vi "Insert Conditional.vi"(8 "error in (no error)":errorcluster, 10 "Insert Conditional":T1, 11 "Test Executive Builder Model in":refnum<class "Test Executive Builder Model.lvclass">) -> (0 "error out":errorcluster, 3 "Test Executive Builder Model out":refnum<class "Test Executive Builder Model.lvclass">, 5 "Unique ID out":string)   [LabVIEW 2017, in "Test Executive Builder Model.lvclass"]
uses:
  Test Executive Builder Model.lvclass
  <vilib>/gpm_packages/@cs/test-executive/Source/Test Executive/TestExecutive Ref/TestExecutive Ref.lvclass
  Test Executive Builder Model Messages/Redraw Tree Msg/Redraw Tree Msg.lvclass
  <vilib>/ActorFramework/Actor/Actor.lvclass
  <vilib>/gpm_packages/@cs/run-time-assertions/Source/Assert/Assert.lvclass
  C:/Program Files (x86)/National Instruments/LabVIEW 2017/vi.lib/ActorFramework/Actor/Actor.lvclass
  Application Dependencies/Insert Conditional.ctl
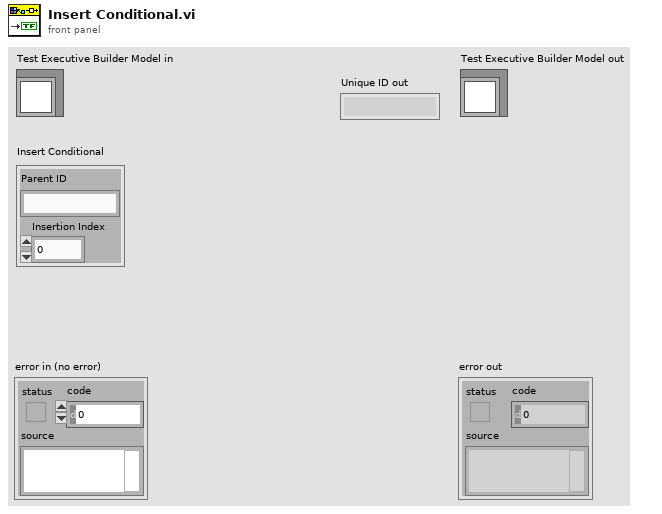
[diagram p1: front panel]
types:
  T1 = typedef "Insert Conditional.ctl" = cluster{"Parent ID":string, "Insertion Index":i32}
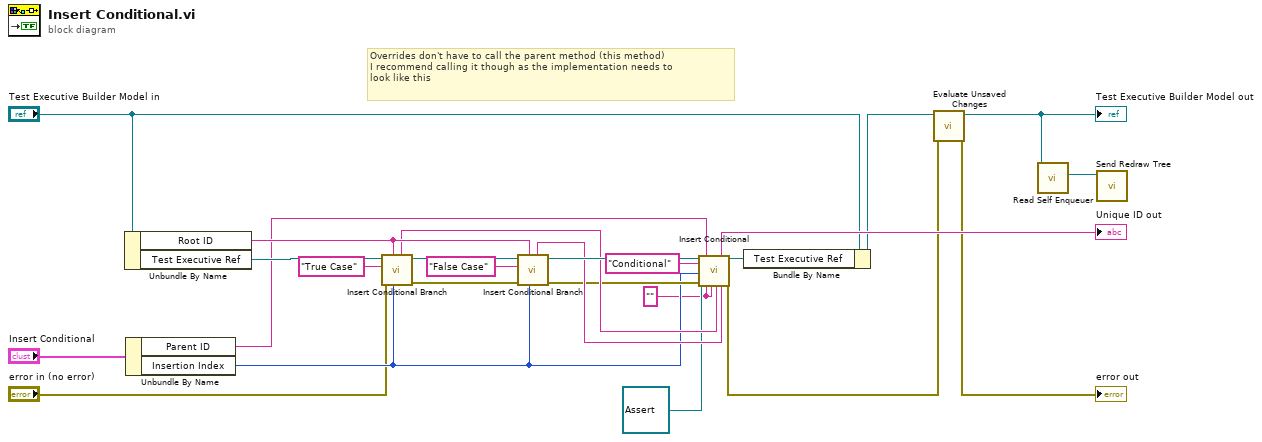
[diagram p0: block diagram]
diagram:
  w5 = "" ("Variable X")
  # "Overrides don't have to call the parent method (this method)\nI recommend calling it though as the implementation needs to\nlook like this"
  n1 = Unbundle By Name("Test Executive Builder Model in") -> ("Root ID"=w21:string, "Test Executive Ref"=w24:refnum<data-value>)
  n2 = Unbundle By Name("Insert Conditional") -> ("Parent ID"=w17:string, "Insertion Index"=w12:i32)
  n3 = call <vilib>:"Insert Conditional Branch.vi"("Insertion Index"=w12, "Parent ID"=w21, "error in (no error)"="error in (no error)", "Name"="True Case", "Test Executive Ref"=w24) -> ("error out"=w20:errorcluster, "Test Executive Ref out"=w19:refnum<data-value>, "Unique ID out"=w15:string)  [unwired: 3 in, 1 out]
  n4 = call <vilib>:"Insert Conditional Branch.vi"("Insertion Index"=w12, "Parent ID"=w21, "error in (no error)"=w20, "Name"="False Case", "Test Executive Ref"=w19) -> ("error out"=w13:errorcluster, "Test Executive Ref out"=w18:refnum<data-value>, "Unique ID out"=w14:string)  [unwired: 3 in, 1 out]
  n5 = call <vilib>:"Insert Conditional.vi"("Test Executive Ref"=w18, "Name"="Conditional", "Insertion Index"=w12, "Assertion"=refnum<class "Assert.lvclass"> refnum, "error in (no error)"=w13, "Parent ID"=w17, "Variable X"=w5, "Variable Y"=w5, "Passing Executive"=w15, "Failing Executive"=w14) -> ("Unique ID out"=→"Unique ID out":string, "Test Executive Ref out"=w9:refnum<data-value>, "error out"=w2:errorcluster)  [unwired: 6 in, 1 out]
  n6 = Bundle By Name(cluster="Test Executive Builder Model in", "Test Executive Ref"=w9) -> (w4:refnum<class "Test Executive Builder Model.lvclass">)
  n7 = call-dynamic "Evaluate Unsaved Changes.vi"("error in (no error)"=w2, "Test Executive Builder Model in"=w4) -> ("error out"=→"error out":errorcluster, "Test Executive Builder Model out"=w3:refnum<class "Test Executive Builder Model.lvclass">)  [unwired: 8 in]
  "Test Executive Builder Model out" <- w3
  n8 = call <vilib>:"Read Self Enqueuer.vi"("Actor"=w3) -> ("Self Enqueuer"=w7:refnum<class "Message Enqueuer.lvclass">)  [unwired: 10 in]
  n9 = call "Send Redraw Tree.vi"("Message Enqueuer"=w7) -> ()  [unwired: 9 in, 2 out]
